vi "RTS Find TCP Socket to Send Too.vi"(8 "Error In":errorcluster, 10 "Server Write Data":string, 11 "Clients":refnum<k5>[](array[refnum])) -> (0 "Error Out":errorcluster, 3 "TCP Send Socket":refnum<k5>)   [LabVIEW 2020]
uses:
  <vilib>/Utility/error.llb/whitespace.ctl
panel:
  out "String Found":string
  out "Numeric":i32
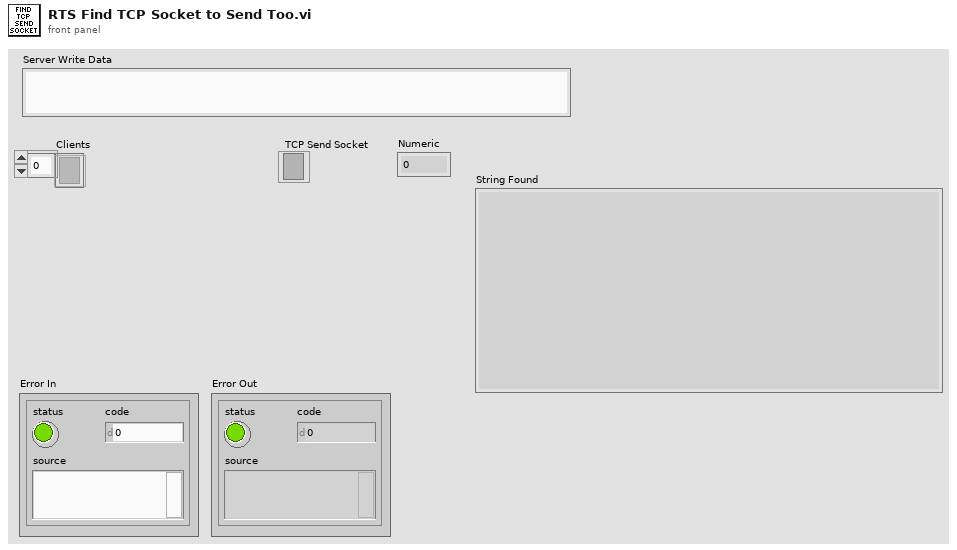
[diagram p1: front panel]
types:
  T1 = typedef "whitespace.ctl" = u16
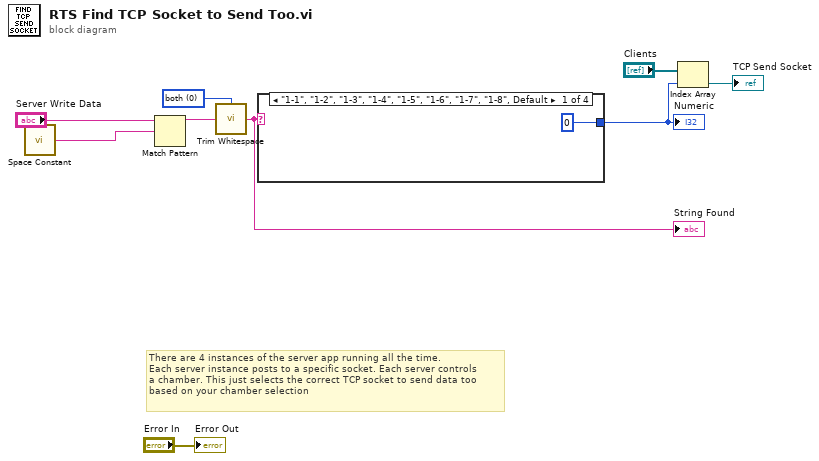
[diagram p0: block diagram]
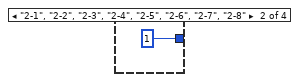
[diagram p2: hidden frame]
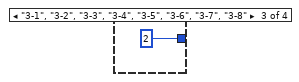
[diagram p3: hidden frame]
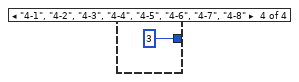
[diagram p4: hidden frame]
diagram:
  w8 = T1 0 items=["both", "start of string", "end of string"] ("location (both)")
  # "There are 4 instances of the server app running all the time. \nEach server instance posts to a specific socket. Each server controls \na chamber. This just selects the correct TCP socket to send data too\nbased on your chamber selection"
  n1 = call <vilib>:"Space Constant.vi"() -> ("String"=w1:string)
  n2 = Match Pattern(string="Server Write Data", regular expression=w1) -> (before substring=w7:string)  [unwired: 1 in, 3 out]
  n3 = call <vilib>:"Trim Whitespace.vi"("string"=w7, "location (both)"=w8) -> ("trimmed string"=w9:string)
  "String Found" <- w9
  n4 = case shown="\"1-1\", \"1-2\", \"1-3\", \"1-4\", \"1-5\", \"1-6\", \"1-7\", \"1-8\", Default" w9 {
    tunnel: [0 1 2 3] -> w4
    frame "1-1", "1-2", "1-3", "1-4", "1-5", "1-6", "1-7", "1-8", Default {
    }
    frame "2-1", "2-2", "2-3", "2-4", "2-5", "2-6", "2-7", "2-8" {
    }
    frame "3-1", "3-2", "3-3", "3-4", "3-5", "3-6", "3-7", "3-8" {
    }
    frame "4-1", "4-2", "4-3", "4-4", "4-5", "4-6", "4-7", "4-8" {
    }
  }
  "Numeric" <- w4
  n5 = Index Array(array="Clients", index=w4) -> (element=→"TCP Send Socket":refnum<k5>)
  "Error Out" <- "Error In"
